vi "Query Multi Eval Meas List Segment SEM Limit Check Results.vi"(6 "Segment (1)":T3=1, 8 "error in (no error)":errorcluster, 9 "Result Type (Current)":i32(ring) items=["Current", "Average"], 10 "Instance (1)":T4=1, 11 "VISA resource name":refnum<visa-resource-name>) -> (0 "error out":errorcluster, 1 "SEM Limit Check Results":T1, 2 "Reliability":T2, 3 "VISA resource name out":refnum<visa-resource-name>, 4 "Expired Statistics":i32, 5 "Out Of Tolerance":i32)   [LabVIEW 2020, in "Rohde&Schwarz CMWXP NR FR1 Measurement.lvlib"]
doc: "Return spectrum emission single value limit check results for segment <no> in list mode.\n\nAttributes:\nRSCMWXPNRFR1M_ATTR_QUERY_MULTI_EVAL_MEAS_LIST_SEGMENT_SEM_CURRENT_LIMIT_CHECK_RESULTS\nRSCMWXPNRFR1M_ATTR_QUERY_MULTI_EVAL_MEAS_LIST_SEGMENT_SEM_AVERAGE_LIMIT_CHECK_RESULTS\n\nRemote-control commands:\nCALCulate:NRSub:MEAS<i>:MEValuation:LIST:SEGMent<no>:SEMask:CURRent?\nCALCulate:NRSub:MEAS<i>:MEValuation:LIST:SEGMent<no>:SEMask:AVERage?"
uses:
  <instrlib>/Rohde&Schwarz CMWXP NR FR1 Measurement/Rohde&Schwarz CMWXP NR FR1 Measurement.lvlib
  <instrlib>/Rohde&Schwarz CMWXP NR FR1 Measurement/Private/_Instance.ctl
  <instrlib>/Rohde&Schwarz CMWXP NR FR1 Measurement/Private/_Segment.ctl
  <instrlib>/Rohde&Schwarz CMWXP NR FR1 Measurement/Private/_SegReliability.ctl
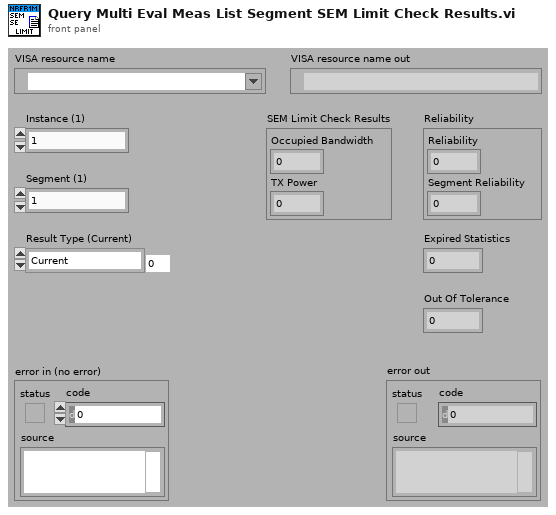
[diagram p1: front panel]
types:
  T1 = cluster{"Occupied Bandwidth":i32, "TX Power":i32}
  T2 = typedef "Rohde&Schwarz CMWXP NR FR1 Measurement.lvlib/_SegReliability.ctl" = cluster{"Reliability":i32, "Segment Reliability":i32}
  T3 = typedef "Rohde&Schwarz CMWXP NR FR1 Measurement.lvlib/_Segment.ctl" = i32
  T4 = typedef "Rohde&Schwarz CMWXP NR FR1 Measurement.lvlib/_Instance.ctl" = i32
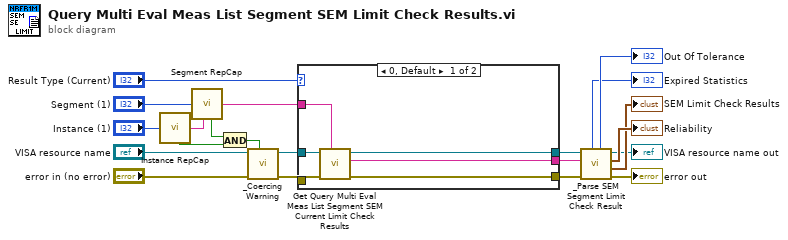
[diagram p0: block diagram]
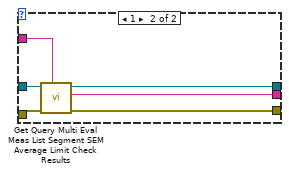
[diagram p2: hidden frame]
diagram:
  n1 = call <instrlib>:"Instance RepCap.vi"("Instance In"="Instance (1)") -> ("In Range?"=w16:bool, "RepCap Identifier Out"=w15:string)  [unwired: 1 in]
  n2 = call <instrlib>:"Segment RepCap.vi"("Segment In"="Segment (1)", "RepCap String In (\"\")"=w15) -> ("In Range?"=w14:bool, "RepCap Identifier Out"=w13:string)
  n3 = And(x=w14, y=w16) -> (x .and. y?=w17:bool)
  n4 = call <instrlib>:"_Coercing Warning.vi"("In Range?"=w17, "error in (no error)"="error in (no error)", "VISA resource name"="VISA resource name") -> ("error out"=w11:errorcluster, "VISA resource name out"=w12:refnum<visa-resource-name>)  [unwired: 7 in]
  n5 = case shown="0, Default" "Result Type (Current)" {
    tunnel: w13 -> [w27 w33]
    tunnel: w12 -> [w26 w32]
    tunnel: w11 -> [w25 w31]
    tunnel: [w24 w30] -> w7
    tunnel: [w23 w29] -> w8
    tunnel: [w22 w28] -> w9
    frame 0, Default {
      n6 = call "Get Query Multi Eval Meas List Segment SEM Current Limit Check Results"("Repeated Capabilities"=w27, "error in (no error)"=w25, "instrument handle"=w26) -> ("error out"=w22:errorcluster, "Query Multi Eval Meas List Segment SEM Current Limit Check Results"=w23:string, "instrument handle out"=w24:refnum<visa-resource-name>)  [unwired: 6 in]
    }
    frame 1 {
      n7 = call "Get Query Multi Eval Meas List Segment SEM Average Limit Check Results"("Repeated Capabilities"=w33, "error in (no error)"=w31, "instrument handle"=w32) -> ("error out"=w28:errorcluster, "Query Multi Eval Meas List Segment SEM Average Limit Check Results"=w29:string, "instrument handle out"=w30:refnum<visa-resource-name>)  [unwired: 6 in]
    }
  }
  n8 = call <instrlib>:"_Parse SEM Segment Limit Check Result.vi"("error in (no error)"=w9, "Input String"=w8, "VISA resource name"=w7) -> ("error out"=→"error out":errorcluster, "SEM Limit Check Results"=→"SEM Limit Check Results":T1, "Reliability Results"=→"Reliability":T2, "VISA resource name out"=→"VISA resource name out":refnum<visa-resource-name>, "Out Of Tolerance"=→"Out Of Tolerance":i32, "Statistic Expired"=→"Expired Statistics":i32)  [unwired: 3 in]
